vi "LoadClassFromName.vi"(8 "error in (no error)":errorcluster, 11 "iClassLoader in":refnum<class "iClassLoader.lvclass">) -> (0 "error out":errorcluster, 3 "iClassLoader out":refnum<class "iClassLoader.lvclass">)   [LabVIEW 2020, in "ClassLoader.lvlib" / "iClassLoader.lvclass"]
uses:
  iClassLoader.lvclass
  ClassLoader_lib/ClassLoader_lib.lvclass
panel:
  in  "AdditionalData":variant
  in  "Class":string
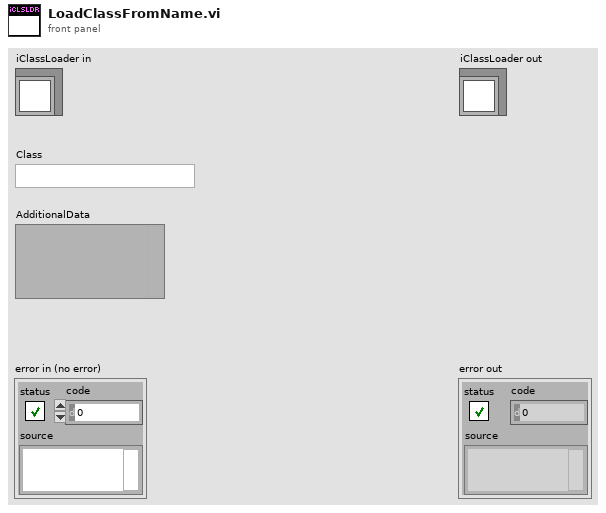
[diagram p1: front panel]
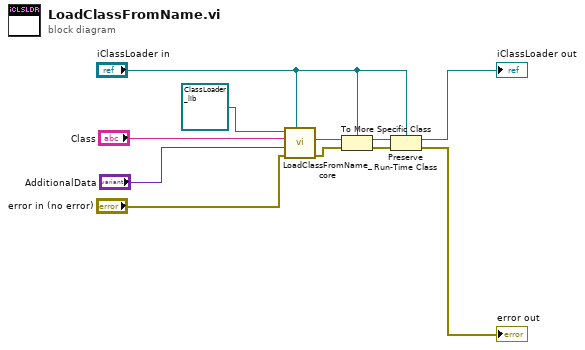
[diagram p0: block diagram]
diagram:
  n1 = call-dynamic "LoadClassFromName_core.vi"("ClassTemplate"="iClassLoader in", "error in (no error)"="error in (no error)", "AdditionalData"="AdditionalData", "Class"="Class", "DLMapper in"=refnum<class "ClassLoader_lib.lvclass"> refnum ("ClassLoader.lvlib:ClassLoader_lib.lvclass")) -> ("error out"=w7:errorcluster, "Class"=w8:refnum<class>)  [unwired: 4 in, 1 out]
  n2 = To More Specific Class(target class="iClassLoader in", reference=w8, error in=w7) -> (specific class reference=w3:refnum<class "iClassLoader.lvclass">, error out=w6:errorcluster)
  n3 = Preserve Run-Time Class(object in=w3, error in=w6, 2:"iClassLoader in") -> (object out=→"iClassLoader out":refnum<class "iClassLoader.lvclass">, error out=→"error out":errorcluster)
